vi "PKG_IMC_GetADchNum.vi"(11 "type":u32) -> (3 "function return":i32)   [LabVIEW 2011, in "IMC_Pkg4xxx.lvlib"]
doc: "PKG_IMC_GetADchNum(unsigned int type);"
uses:
  IMC_Pkg4xxx.lvlib
  IMC_Pkg4xxx.dll
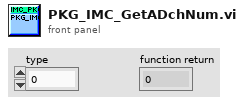
[diagram p1: front panel]
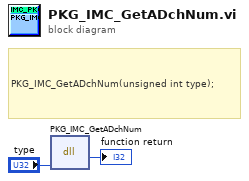
[diagram p0: block diagram]
diagram:
  # "PKG_IMC_GetADchNum(unsigned int type);"
  n1 = dll-call lib="PTH1mabs F光盘刻录\niMC MotionIMCNet_V4.0IMCAppincLabviewIMC_PKG4xxxIMC_PKG4xxx\nIMC_Pkg4xxx.*" fn="PKG_IMC_GetADchNum"("type"="type") -> (→"function return":i32)  [unwired: 4 in, 2 out]
